vi "Read custom data.vi"(8 "error in":errorcluster, 10 "Key":string="awefawe", 11 "Image":T1) -> (0 "error out":errorcluster, 1 "Custom Data Out":string, 3 "Image (duplicate)":T1)   [LabVIEW 2013]
doc: "This .vi runs IMAQ Read Key. It retries several times if the key doesn't exist. If it fails, then it returns the error with the calling .vi's name and the key that was missing."
uses:
  <vilib>/vision/Image Controls.llb/IMAQ Image.ctl
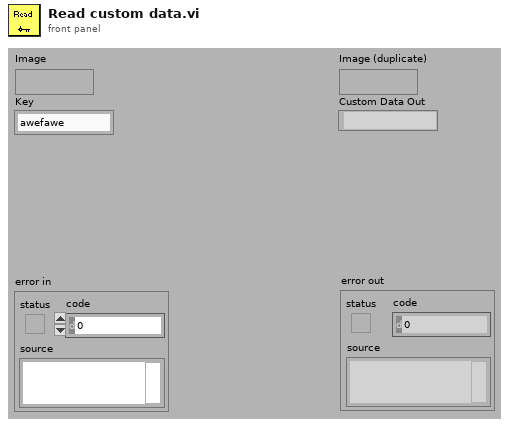
[diagram p1: front panel]
types:
  T1 = typedef "IMAQ Image.ctl" = refnum<image>
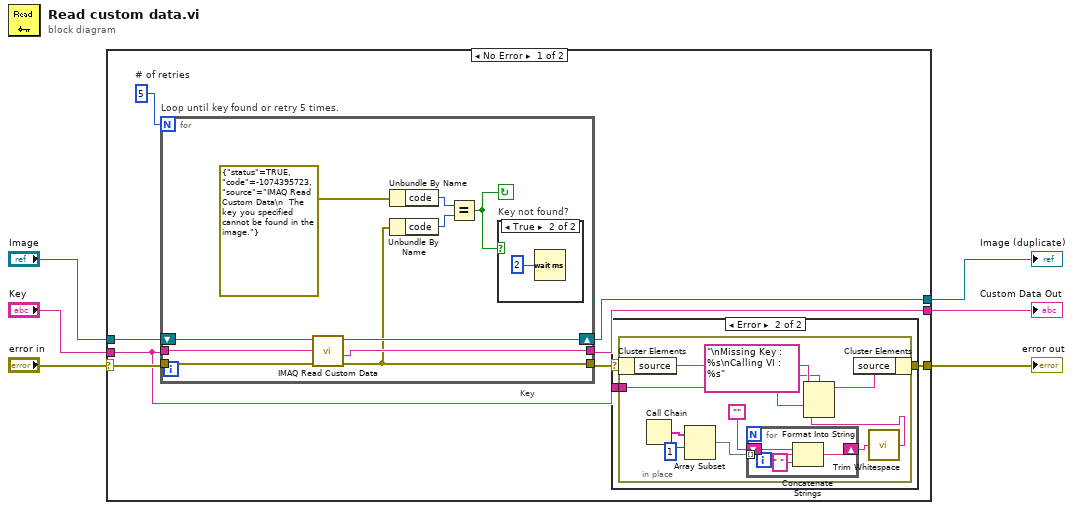
[diagram p0: block diagram]
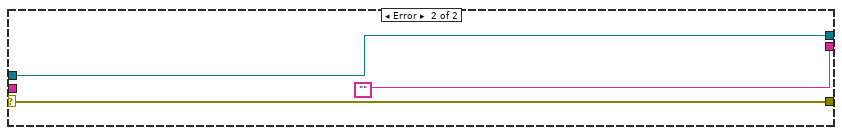
[diagram p4: hidden frame]
diagram:
  n1 = case shown="No Error" "error in" {
    selector: "error in" -> [w10 w46]
    tunnel: [w8 w46] -> w6
    tunnel: "Image" -> [w14 w45]
    tunnel: [w13 w45] -> w4
    tunnel: [w12 ""] -> w3
    tunnel: "Key" -> [w7 _]
    frame No Error {
      w11 = 5  # # of retries
      # "Key"
      n2 = for "Loop until key found or retry 5 times." {
        N: w11 -> [_]
        shift-right: [w39] -> w13
        shift-left: w14 -> [w40]
        tunnel: [w38] -> w12
        tunnel: w7 -> [w37]
        tunnel: w10 -> [w41]
        tunnel: [w36] -> w9
        stop <- w33 continue-if-true
        n3 = call "IMAQ Read Custom Data"("error in (no error)"=w41, "Key"=w37, "Image"=w40) -> ("error out"=w36:errorcluster, "Custom Data Out"=w38:string, "Image (duplicate)"=w39:T1)  [unwired: 1 in, 5 out]
        n4 = Unbundle By Name(errorcluster {"status"=TRUE, "code"=-1074395723, "source"="IMAQ Read Custom Data\n  The key you specified cannot be found in the image."} ("error out")) -> ("code"=w34:i32)
        n5 = Unbundle By Name(w36) -> ("code"=w35:i32)
        n6 = Equal?(x=w34, y=w35) -> (x = y?=w33:bool)
        n7 = case "Key not found?" shown="True" w33 {
          frame False {
          }
          frame True {
            n8 = Wait (ms)(milliseconds to wait=u32 2) -> ()  [unwired: 1 out]
          }
        }
      }
      n9 = case shown="Error" w9 {
        selector: w9 -> [w15 w18]
        tunnel: [w15 w16] -> w8
        tunnel: w7 -> [_ w17]
        frame No Error {
        }
        frame Error {
          n10 = in-place {
            in-place-border: w17 -> [w24]
            n11 = in-place-cluster #1(w18) -> ("source"=w26:string)
            n12 = Call Chain() -> (call chain=w27:string[])
            n13 = Array Subset(array=w27, index=1) -> (w22:string[])  [unwired: 1 in]
            n14 = for {
              tunnel: w22 -> [w32] mode=indexing
              shift-right: [w30] -> w20
              shift-left: "" -> [w29]
              n15 = Concatenate Strings(w29, w32, " " ("string")) -> (w30:string)
            }
            n16 = call <vilib>:"Trim Whitespace.vi"("string"=w20) -> ("trimmed string"=w19:string)  [unwired: 1 in]
            n17 = Format Into String(format string="\nMissing Key : %s\nCalling VI : %s", initial string=w26, w24, w19) -> (resulting string=w25:string)  [unwired: 1 in, 1 out]
            n18 = in-place-cluster #1("source"=w25) -> (w16:errorcluster)
          }
        }
      }
    }
    frame Error {
    }
  }
  "error out" <- w6
  "Image (duplicate)" <- w4
  "Custom Data Out" <- w3
